vi "SMC_Close.vi"(8 "error in (no error)":errorcluster) -> (0 "error out":errorcluster)   [LabVIEW 2015]
uses:
  SubVIs/JS_Comm.llb/Communication_Job.ctl
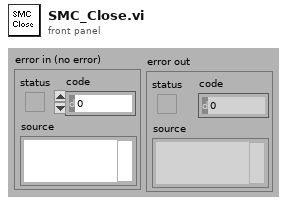
[diagram p1: front panel]
types:
  T1 = typedef "Communication_Job.ctl" = enum16{"Init", "Read", "hasLF", "Get1Line", "Write", "Close", "Clear"}
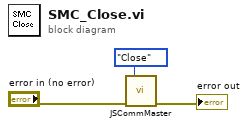
[diagram p0: block diagram]
diagram:
  n1 = call "JSCommMaster.vi"("CommJob"=Communication_Job."Close", "error in (no error)"="error in (no error)") -> ("error out"=→"error out":errorcluster)  [unwired: 11 in, 2 out]
